vi "SetCoodinateSystem.vi"(8 "error in":errorcluster, 9 "ROI Descriptor":T2 {"Contours"."Type" items=["No Selection", "Point", "Line", "Rectangle", "Oval", "Polygon", "Free", "Annulus", "Unused2", "Unused3", "Broken Line", "Free Hand Line", "Rotated Rectangle"]}, 10 "ROI1":T1, 11 "Refnum in":T5) -> (0 "error out":errorcluster, 1 "Image Out":T5(plugin-control), 3 "Coordinate System":T6)   [LabVIEW 2019, in "Algorithm.lvclass"]
uses:
  FrameworkOverrides/Algorithm.lvclass
  <vilib>/vision/NI_Vision_Development_Module.lvlib
  <vilib>/vision/Image Controls.llb/IMAQ Image.ctl
panel:
  out "Base Points Cluster":T4 {"Array to two Parallel Lines"."Contours"."Type" items=["No Selection", "Point", "Line", "Rectangle", "Oval", "Polygon", "Freehand Region", "Annulus", "Unused2", "Unused3", "Broken Line", "Freehand Line", "Rotated Rectangle"]; "Circle Roi"."Contours"."Type" items=["No Selection", "Point", "Line", "Rectangle", "Oval", "Polygon", "Freehand Region", "Annulus", "Unused2", "Unused3", "Broken Line", "Freehand Line", "Rotated Rectangle"]}
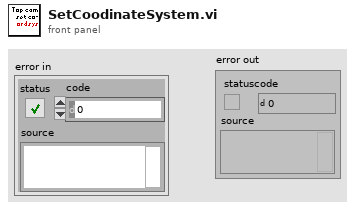
[diagram p1: front panel]
types:
  T1 = cluster{"ROI":cluster{"Left":i32, "Top":i32, "Right":i32, "Bottom":i32, "Rotation":dbl}, "EdgeOptions":cluster{"EdgePolarity":i32, "KernelSize":i32, "Width":i32, "MinimumEdgeStrength":i32, "InterpolationType":i32, "DataProcessingMethod":i32}, "LineOptions":cluster{"NumberofLines":i32, "Type":i32, "MinScore":i32, "MaxScore":i32, "Orientation":i32, "AngleRange":i32, "AngleTolerance":i32, "StepSize":i32, "MinSNR":i32, "MinPoints":i32, "HoughIterations":i32}, "Process":i32, "StepSize":i32, "SearchDirection":i32, "CircleEdgeOptions":cluster{"SearchDirection":i32, "EdgeOptions":cluster{"EdgePolarity":i32, "KernelSize":i32, "Width":i32, "MinimumEdgeStrength":i32, "InterpolationType":i32, "DataProcessingMethod":i32}}, "CircleFitOptions":cluster{"Process":i32, "StepSize":i32, "MAxPixelRadius":i32}, "CircleSearchDirection":i32, "CurveParameters":cluster{"ExtractionMode":i32, "EdgeThreshold":i32, "EdgeFilterSize":i32, "MinLength":i32, "RowSearchStepSize":i32, "ColSearchStepSize":i32, "MaxEndpointGap":i32, "Closed":bool, "Subpixel":bool}, "MinimumMatchScore":i32, "CircleDescriptor":cluster{"MinRadius":i32, "MaxRadius":i32}, "EllipseDescriptor":cluster{"MinMajorRadius":i32, "MaxMajorRadius":i32, "MinMinorRadius":i32, "MaxMinorRadius":i32}, "ParallelLines":cluster{"First":i32, "Second":i32, "Third":i32}}
  T2 = cluster{"Global Rectangle":i32[], "Contours":cluster{"ID":enum32{"External", "Internal"}, "Type":u32, "Coordinates":i32[]}[]}
  T3 = typedef "ROI Descriptor" = cluster{"Global Rectangle":i32[], "Contours":cluster{"ID":enum32{"External", "Internal"}, "Type":u32, "Coordinates":i32[]}[]}
  T4 = cluster{"Array to two Parallel Lines":T3[], "Circle Roi":T3, "Perpendicular Line ":cluster{"Point 2":cluster{"X":sgl, "Y":sgl}, "Point 1":cluster{"X":sgl, "Y":sgl}}, "Staright Edges Of Co ordinate":cluster{"Point1 (Pixels)":cluster{"X":sgl, "Y":sgl}, "Point2 (Pixels)":cluster{"X":sgl, "Y":sgl}}}
  T5 = typedef "IMAQ Image.ctl" = refnum<image>
  T6 = cluster{"Origin":cluster{"X":sgl, "Y":sgl}, "Angle (deg)":sgl, "Axis Reference":u32}
  T7 = typedef "IMAQ Line" = cluster{"Start X":i32, "Start Y":i32, "End X":i32, "End Y":i32}
  T8 = enum16{"Get First Edge", "Get First + Last Edge", "Get All Edges", "Get Best Edge"}
  T9 = cluster{"EdgePolarity":i32, "KernelSize":i32, "Width":i32, "MinimumEdgeStrength":i32, "InterpolationType":i32, "DataProcessingMethod":i32}
  T10 = cluster{"SearchDirection":i32, "EdgeOptions":cluster{"EdgePolarity":i32, "KernelSize":i32, "Width":i32, "MinimumEdgeStrength":i32, "InterpolationType":i32, "DataProcessingMethod":i32}}
  T11 = cluster{"NumberofLines":i32, "Type":i32, "MinScore":i32, "MaxScore":i32, "Orientation":i32, "AngleRange":i32, "AngleTolerance":i32, "StepSize":i32, "MinSNR":i32, "MinPoints":i32, "HoughIterations":i32}
  T12 = cluster{"Point1 (Pixels)":cluster{"X":sgl, "Y":sgl}, "Point2 (Pixels)":cluster{"X":sgl, "Y":sgl}, "Point1 (Real-World)":cluster{"X":sgl, "Y":sgl}, "Point2 (Real-World)":cluster{"X":sgl, "Y":sgl}, "Angle (Pixel)":dbl, "Angle (Real-World)":dbl, "Score":dbl, "Straightness":dbl, "Average SNR (db)":dbl, "Calibration Valid":bool}[]
  T13 = typedef "Search Line.ctl" = cluster{"Start Point":cluster{"X":sgl, "Y":sgl}, "End Point":cluster{"X":sgl, "Y":sgl}, "Edge Info":T14[], "Edge Map":dbl[], "Calibration Valid":bool}
  T14 = typedef "Edge New.ctl" = cluster{"Location (Pixel)":cluster{"X":sgl, "Y":sgl}, "Location (Real-World)":cluster{"X":sgl, "Y":sgl}, "Distance (Pixel)":dbl, "Distance (Real-World)":dbl, "Strength":dbl, "Noise":dbl, "Rising?":bool}
  T15 = cluster{"Point1 (Pixels)":cluster{"X":sgl, "Y":sgl}, "Point2 (Pixels)":cluster{"X":sgl, "Y":sgl}, "Point1 (Real-World)":cluster{"X":sgl, "Y":sgl}, "Point2 (Real-World)":cluster{"X":sgl, "Y":sgl}, "Angle (Pixel)":dbl, "Angle (Real-World)":dbl, "Score":dbl, "Straightness":dbl, "Average SNR (db)":dbl, "Calibration Valid":bool}
  T16 = cluster{"Point1 (Pixels)":cluster{"X":sgl, "Y":sgl}, "Point2 (Pixels)":cluster{"X":sgl, "Y":sgl}}
  T17 = cluster{"ROI Descriptor":T3, "ROI Descriptor":T3, "ROI Descriptor":T3}
  T18 = cluster{"Location (Pixel)":cluster{"X":sgl, "Y":sgl}, "Location (Pixel)":cluster{"X":sgl, "Y":sgl}, "Location (Pixel)":cluster{"X":sgl, "Y":sgl}}
  T19 = cluster{"Center":cluster{"X":sgl, "Y":sgl}, "Radius":dbl}
  T20 = cluster{"Point 1":cluster{"X":sgl, "Y":sgl}, "Point 2":cluster{"X":sgl, "Y":sgl}}
  T21 = cluster{"Point 2":cluster{"X":sgl, "Y":sgl}, "Point 1":cluster{"X":sgl, "Y":sgl}}
  T22 = cluster{"Point 2":cluster{"X":sgl, "Y":sgl}, "Point 1":cluster{"X":sgl, "Y":sgl}, "Point1 (Pixels)":cluster{"X":sgl, "Y":sgl}}
  T23 = cluster{"X":sgl, "Y":sgl, "Y":sgl, "Radius":dbl, "Y":sgl, "Radius":dbl}
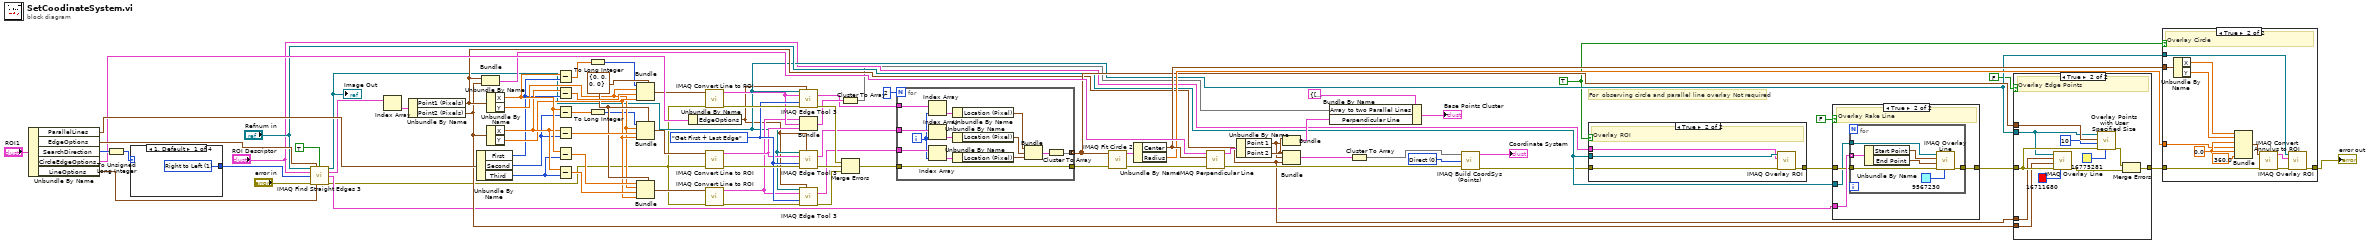
[diagram p0: block diagram]
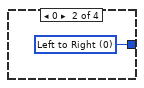
[diagram p6: hidden frame]
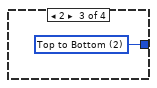
[diagram p7: hidden frame]
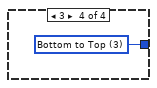
[diagram p8: hidden frame]
diagram:
  w13 = TRUE ("Boolean")
  w50 = T7 {"Start X"=0, "Start Y"=0, "End X"=0, "End Y"=0} ("Line")
  w58 = u32 0 items=["Direct", "Indirect"] ("Axis Reference")
  w29 = T8."Get First + Last Edge" ("Process")
  # "For  observing circle and parallel line overlay Not required"
  n1 = Unbundle By Name("ROI1") -> ("ParallelLines"=w82:cluster{"First":i32, "Second":i32, "Third":i32}, "EdgeOptions"=w81:T9, "SearchDirection"=w80:i32, "CircleEdgeOptions"=w79:T10, "LineOptions"=w78:T11)
  n2 = To Unsigned Long Integer(number=w80) -> (unsigned 32bit integer=w27:u32)
  n3 = case shown="1, Default" w27 {
    tunnel: [w83 w84 w85 w86] -> w28
    frame 1, Default {
      w83 = u32 1 items=["Left to Right", "Right to Left", "Top to Bottom", "Bottom to Top"] ("Search Direction")
    }
    frame 0 {
      w84 = u32 0 items=["Left to Right", "Right to Left", "Top to Bottom", "Bottom to Top"] ("Search Direction")
    }
    frame 2 {
      w85 = u32 2 items=["Left to Right", "Right to Left", "Top to Bottom", "Bottom to Top"] ("Search Direction")
    }
    frame 3 {
      w86 = u32 3 items=["Left to Right", "Right to Left", "Top to Bottom", "Bottom to Top"] ("Search Direction")
    }
  }
  n4 = call "IMAQ Find Straight Edges 3"("Image"="Refnum in", "Edge Options"=w81, "Optimized Mode"=TRUE, "ROI Descriptor"="ROI Descriptor", "Search Direction"=w28, "error in (no error)"="error in", "Line Options"=w78) -> ("Image (duplicate)"=w15:T5, "Straight Edges"=w76:T12, "Search Lines Information"=w21:T13[], "error out"=w4:errorcluster)  [unwired: 4 in, 1 out]
  "Image Out" <- w15
  n5 = Index Array(array=w76) -> (element=w68:T15)  [unwired: 1 in]
  n6 = Unbundle By Name(w68) -> ("Point1 (Pixels)"=w23:cluster{"X":sgl, "Y":sgl}, "Point2 (Pixels)"=w22:cluster{"X":sgl, "Y":sgl})
  n7 = Unbundle By Name(w82) -> ("First"=w37:i32, "Second"=w36:i32, "Third"=w35:i32)
  n8 = Bundle("Point1 (Pixels)"=w23, "Point2 (Pixels)"=w22) -> (w32:T16)  [unwired: 1 in]
  n9 = Unbundle By Name(w23) -> ("X"=w49:sgl, "Y"=w44:sgl)
  n10 = Unbundle By Name(w22) -> ("X"=w47:sgl, "Y"=w45:sgl)
  n11 = Subtract(x=w49, y=w37) -> (x-y=w74:sgl)
  n12 = Subtract(x=w47, y=w37) -> (x-y=w73:sgl)
  n13 = Subtract(x=w49, y=w36) -> (x-y=w72:sgl)
  n14 = Subtract(x=w47, y=w36) -> (x-y=w71:sgl)
  n15 = Subtract(x=w49, y=w35) -> (x-y=w48:sgl)
  n16 = Subtract(x=w47, y=w35) -> (x-y=w46:sgl)
  n17 = To Long Integer(number=w74) -> (32bit integer=w31:i32)
  n18 = To Long Integer(number=w72) -> (32bit integer=w30:i32)
  n19 = Bundle(cluster=w50, "Start X"=w31, "Start Y"=w44, "End X"=w73, "End Y"=w45) -> (w56:T7)
  n20 = Bundle(cluster=w50, "Start X"=w30, "Start Y"=w44, "End X"=w71, "End Y"=w45) -> (w55:T7)
  n21 = Bundle(cluster=w50, "Start X"=w48, "Start Y"=w44, "End X"=w46, "End Y"=w45) -> (w51:T7)
  n22 = Unbundle By Name(w79) -> ("EdgeOptions"=w14:T9)
  n23 = call "IMAQ Convert Line to ROI"("error in (no error)"=w4, "Line"=w56) -> ("error out"=w64:errorcluster, "ROI Descriptor"=w18:T3)  [unwired: 7 in]
  n24 = call "IMAQ Convert Line to ROI"("error in (no error)"=w4, "Line"=w55) -> ("error out"=w63:errorcluster, "ROI Descriptor"=w17:T3)  [unwired: 7 in]
  n25 = call "IMAQ Convert Line to ROI"("error in (no error)"=w4, "Line"=w51) -> ("error out"=w52:errorcluster, "ROI Descriptor"=w16:T3)  [unwired: 7 in]
  n26 = call "IMAQ Edge Tool 3"("Image"=w15, "Edge Options"=w14, "ROI Descriptor"=w18, "Process"=w29, "error in (no error)"=w64) -> ("Edge Information"=w39:T14[], "error out"=w65:errorcluster)  [unwired: 6 in, 3 out]
  n27 = Bundle("ROI Descriptor"=w16, "ROI Descriptor"=w18, "ROI Descriptor"=w17) -> (w40:T17)  [unwired: 1 in]
  n28 = call "IMAQ Edge Tool 3"("Image"=w15, "Edge Options"=w14, "ROI Descriptor"=w17, "Process"=w29, "error in (no error)"=w63) -> ("Edge Information"=w38:T14[], "error out"=w66:errorcluster)  [unwired: 6 in, 3 out]
  n29 = call "IMAQ Edge Tool 3"("Image"=w15, "Edge Options"=w14, "ROI Descriptor"=w16, "Process"=w29, "error in (no error)"=w52) -> ("Edge Information"=w41:T14[], "error out"=w43:errorcluster)  [unwired: 6 in, 3 out]
  n30 = Cluster To Array(cluster=w40) -> (array=w8:T3[])
  n31 = Merge Errors(w65, w66, w43) -> (w60:errorcluster)
  n32 = for {
    N: 2 -> [_]
    tunnel: w39 -> [w96]
    tunnel: w38 -> [w94]
    tunnel: [w87] -> w24 mode=concatenating
    tunnel: [w99] -> w7
    tunnel: w60 -> [w99]
    tunnel: w41 -> [w98]
    i -> [w93]
    n33 = Index Array(array=w96, index=w93) -> (element=w95:T14)
    n34 = Index Array(array=w94, index=w93) -> (element=w92:T14)
    n35 = Index Array(array=w98, index=w93) -> (element=w97:T14)
    n36 = Unbundle By Name(w95) -> ("Location (Pixel)"=w91:cluster{"X":sgl, "Y":sgl})
    n37 = Unbundle By Name(w92) -> ("Location (Pixel)"=w90:cluster{"X":sgl, "Y":sgl})
    n38 = Unbundle By Name(w97) -> ("Location (Pixel)"=w88:cluster{"X":sgl, "Y":sgl})
    n39 = Bundle("Location (Pixel)"=w91, "Location (Pixel)"=w90, "Location (Pixel)"=w88) -> (w89:T18)  [unwired: 1 in]
    n40 = Cluster To Array(cluster=w89) -> (array=w87:cluster{"X":sgl, "Y":sgl}[])
  }
  n41 = call "IMAQ Fit Circle 2"("error in (no error)"=w7, "Radial Points"=w24) -> ("error out"=w6:errorcluster, "Circle"=w53:T19)  [unwired: 4 in, 4 out]
  n42 = Unbundle By Name(w53) -> ("Center"=w26:cluster{"X":sgl, "Y":sgl}, "Radius"=w25:dbl)
  n43 = call "IMAQ Perpendicular Line"("error in (no error)"=w6, "Point"=w26, "Line"=w32) -> ("error out"=w59:errorcluster, "Perpendicular Line"=w77:T20)  [unwired: 6 in, 1 out]
  n44 = Unbundle By Name(w77) -> ("Point 1"=w61:cluster{"X":sgl, "Y":sgl}, "Point 2"=w62:cluster{"X":sgl, "Y":sgl})
  n45 = Bundle("Point 2"=w62, "Point 1"=w61) -> (w69:T21)  [unwired: 1 in]
  n46 = Bundle("Point 2"=w62, "Point 1"=w61, "Point1 (Pixels)"=w23) -> (w57:T22)  [unwired: 1 in]
  n47 = Bundle By Name(cluster=T4 {"Array to two Parallel Lines"=[], "Circle Roi"={"Global Rectangle"=[], "Contours"=[]}, "Perpendicular Line "={"Point 2"={"X"=0.0, "Y"=0.0}, "Point 1"={"X"=0.0, "Y"=0.0}}, "Staright Edges Of Co ordinate"={"Point1 (Pixels)"={"X"=0.0, "Y"=0.0}, "Point2 (Pixels)"={"X"=0.0, "Y"=0.0}}}, "Array to two Parallel Lines"=w8, "Perpendicular Line"=w69) -> (→"Base Points Cluster":T4)
  n48 = Cluster To Array(cluster=w57) -> (array=w54:cluster{"X":sgl, "Y":sgl}[])
  n49 = call "IMAQ Build CoordSys (Points)"("Reference Points"=w54, "Axis Reference"=w58, "error in (no error)"=w59) -> ("Coordinate System"=→"Coordinate System":T6, "error out"=w2:errorcluster)  [unwired: 2 in]
  n50 = case shown="True" w13 {
    tunnel: "Refnum in" -> [_ w104]
    tunnel: "ROI Descriptor" -> [_ w103]
    tunnel: w2 -> [w100 w102]
    tunnel: [w100 w101] -> w20
    frame False {
    }
    frame True {
      # "Overlay ROI"
      n51 = call "IMAQ Overlay ROI"("error in (no error)"=w102, "ROI Descriptor"=w103, "Image"=w104) -> ("error out"=w101:errorcluster)  [unwired: 7 in, 1 out]
    }
  }
  n52 = case shown="True" FALSE ("Boolean 2") {
    tunnel: w21 -> [_ w109]
    tunnel: w20 -> [w105 w108]
    tunnel: [w105 w107] -> w3
    tunnel: "Refnum in" -> [_ w106]
    frame False {
    }
    frame True {
      # "Overlay Rake Line"
      n53 = for {
        tunnel: w109 -> [w116] mode=indexing
        tunnel: w108 -> [w113]
        tunnel: [w112] -> w107
        tunnel: w106 -> [w111]
        n54 = Unbundle By Name(w116) -> ("Start Point"=w115:cluster{"X":sgl, "Y":sgl}, "End Point"=w114:cluster{"X":sgl, "Y":sgl})
        n55 = call "IMAQ Overlay Line"("Color"=u32 9567230, "error in (no error)"=w113, "End Point"=w114, "Start Point"=w115, "Image"=w111) -> ("error out"=w112:errorcluster)  [unwired: 5 in, 1 out]
      }
    }
  }
  n56 = case shown="True" FALSE ("Boolean 3") {
    tunnel: w24 -> [_ w128]
    tunnel: w3 -> [w117 w122]
    tunnel: [w117 w123] -> w5
    tunnel: w23 -> [_ w121]
    tunnel: w22 -> [_ w120]
    tunnel: w15 -> [_ w119]
    frame False {
    }
    frame True {
      # "Overlay Edge Points"
      n57 = call "IMAQ Overlay Line"("Color"=u32 16711680, "error in (no error)"=w122, "End Point"=w120, "Start Point"=w121, "Image"=w119) -> ("error out"=w124:errorcluster)  [unwired: 5 in, 1 out]
      n58 = call "Overlay Points with User Specified Size.vi"("Color"=u32 16775281, "error in"=w122, "Point Diameter (5)"=u32 10, "Points"=w128, "Image In"=w119) -> ("error out"=w125:errorcluster)  [unwired: 5 in, 1 out]
      n59 = Merge Errors(w125, w124) -> (w123:errorcluster)
    }
  }
  n60 = case shown="True" w13 {
    tunnel: w26 -> [_ w138]
    tunnel: w25 -> [_ w135]
    tunnel: w15 -> [_ w133]
    tunnel: w5 -> [w129 w132]
    tunnel: [w129 w130] -> w1
    frame False {
    }
    frame True {
      w139 = sgl 0.0 ("Y")
      # "Overlay Circle"
      n61 = Unbundle By Name(w138) -> ("X"=w137:sgl, "Y"=w136:sgl)
      n62 = Bundle("X"=w137, "Y"=w136, "Y"=w139, "Radius"=w135, "Y"=w139, "Radius"=360.0) -> (w141:T23)  [unwired: 1 in]
      n63 = call "IMAQ Convert Annulus to ROI"("error in (no error)"=w132, "Annulus"=w141) -> ("error out"=w131:errorcluster, "ROI Descriptor"=w134:T3)  [unwired: 7 in]
      n64 = call "IMAQ Overlay ROI"("error in (no error)"=w131, "ROI Descriptor"=w134, "Image"=w133) -> ("error out"=w130:errorcluster)  [unwired: 7 in, 1 out]
    }
  }
  "error out" <- w1
